vi "Configure Basic TDD.vi"(0 "VISA resource name":refnum<visa-resource-name>, 1 "TDD Response (0: adRMS)":i32(ring) items=["adRMS", "adQuasiPk", "adPeak"], 2 "Post Filter Gain (0: pfgAuto)":i32(ring) items=["pfgAuto", "pfgdBminus12", "pfgdBminus6", "pfgdB0", "pfgdB6", "pfgdB12", "pfgdB18", "pfgdB24", "pfgdB30", "pfgdB36", "pfgdB42", "pfgdB48", "pfgdB54", "pfgdB60", "pfgdB66"], 5 "Analyzer (0: A0)":i32(ring) items=["A0", "A1"], 7 "Measurement (0: adAmplitude)":i32(ring) items=["adAmplitude", "adRation", "adTHDNAmpe", "adTHDNRatio", "adSINADRatio", "adCrestFactor"], 9 "Detect Rate (0: adFast)":i32(ring) items=["adFast", "adPrecise", "adrps1", "adrps2", "adrps4", "adrps8", "adrps16", "adrps32", "adrps64", "adrps128", "adrps256"], 11 "error in (no error)":errorcluster, 12 "Weighting Filter (0: adNoWt)":i32(ring) items=["adNoWt", "adAWt", "adCMsg", "adCCITT", "adCCIRwtd", "adCCIRunwtd", "adCCIR2kHz"]) -> (4 "VISA resource name out":refnum<visa-resource-name>, 15 "error out":errorcluster)   [LabVIEW 2014, in "Stanford Research SR1.lvlib"]
doc: "Configures the basic attributes for the TDD Analyzer."
uses:
  Stanford Research SR1.lvlib
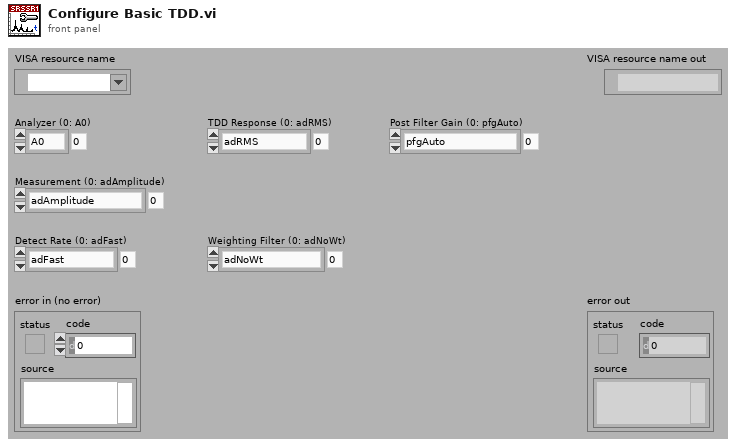
[diagram p1: front panel]
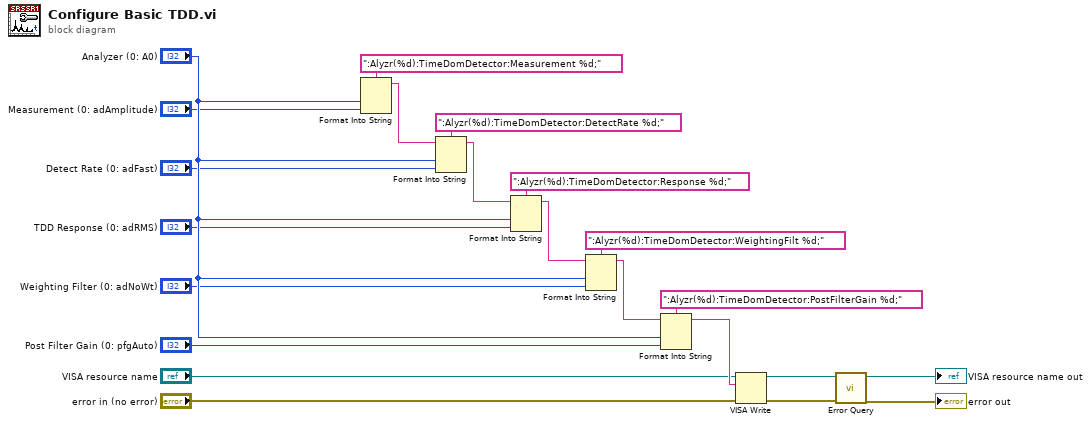
[diagram p0: block diagram]
diagram:
  n1 = Format Into String(format string=":Alyzr(%d):TimeDomDetector:Measurement %d;", "Analyzer (0: A0)", "Measurement (0: adAmplitude)") -> (resulting string=w21:string)  [unwired: 2 in, 1 out]
  n2 = Format Into String(format string=":Alyzr(%d):TimeDomDetector:DetectRate %d;", initial string=w21, "Analyzer (0: A0)", "Detect Rate (0: adFast)") -> (resulting string=w19:string)  [unwired: 1 in, 1 out]
  n3 = Format Into String(format string=":Alyzr(%d):TimeDomDetector:Response %d;", initial string=w19, "Analyzer (0: A0)", "TDD Response (0: adRMS)") -> (resulting string=w17:string)  [unwired: 1 in, 1 out]
  n4 = Format Into String(format string=":Alyzr(%d):TimeDomDetector:WeightingFilt %d;", initial string=w17, "Analyzer (0: A0)", "Weighting Filter (0: adNoWt)") -> (resulting string=w15:string)  [unwired: 1 in, 1 out]
  n5 = Format Into String(format string=":Alyzr(%d):TimeDomDetector:PostFilterGain %d;", initial string=w15, "Analyzer (0: A0)", "Post Filter Gain (0: pfgAuto)") -> (resulting string=w13:string)  [unwired: 1 in, 1 out]
  n6 = VISA Write(VISA resource name="VISA resource name", write buffer=w13, error in (no error)="error in (no error)") -> (VISA resource name out=w10:refnum<visa-resource-name>, error out=w9:errorcluster)  [unwired: 1 out]
  n7 = call "Error Query.vi"("error in (no error)"=w9, "VISA resource name"=w10) -> ("error out"=→"error out":errorcluster, "VISA resource name out"=→"VISA resource name out":refnum<visa-resource-name>)  [unwired: 6 in, 2 out]
